vi "SEA_9811_ARINCword2data.vi"(7 "Reverse label bits (F)":bool, 8 "error in (no error)":errorcluster, 10 "timestamp (DBL) in":dbl, 11 "ARINC word in":T2 format="%032b") -> (0 "error out":errorcluster, 3 "ARINC word out":T1 {"ARINC word" format="%032b"})   [LabVIEW 2015]
uses:
  Typdefs/ARINC word.ctl
  Typdefs/ARINC word cluster.ctl
panel:
  out "number":u8 format="%.0o"
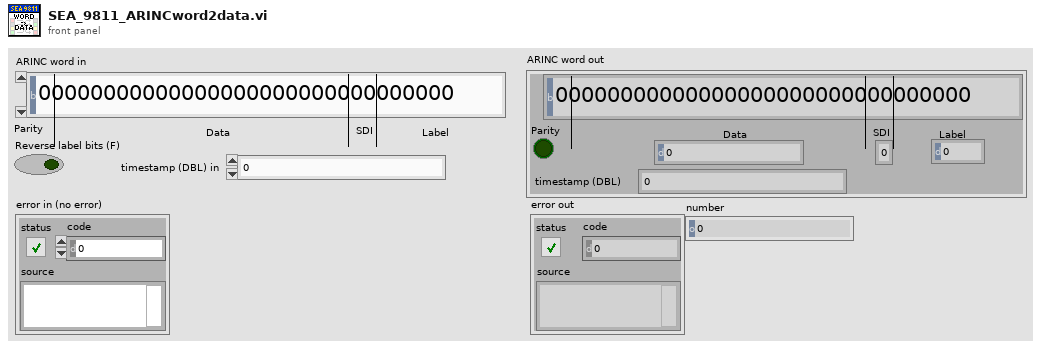
[diagram p1: front panel]
types:
  T1 = typedef "ARINC word cluster.ctl" = cluster{"ARINC word":T2, "Label":u8, "SDI":u8, "Data":u32, "Parity":bool, "timestamp (DBL)":dbl}
  T2 = typedef "ARINC word.ctl" = u32
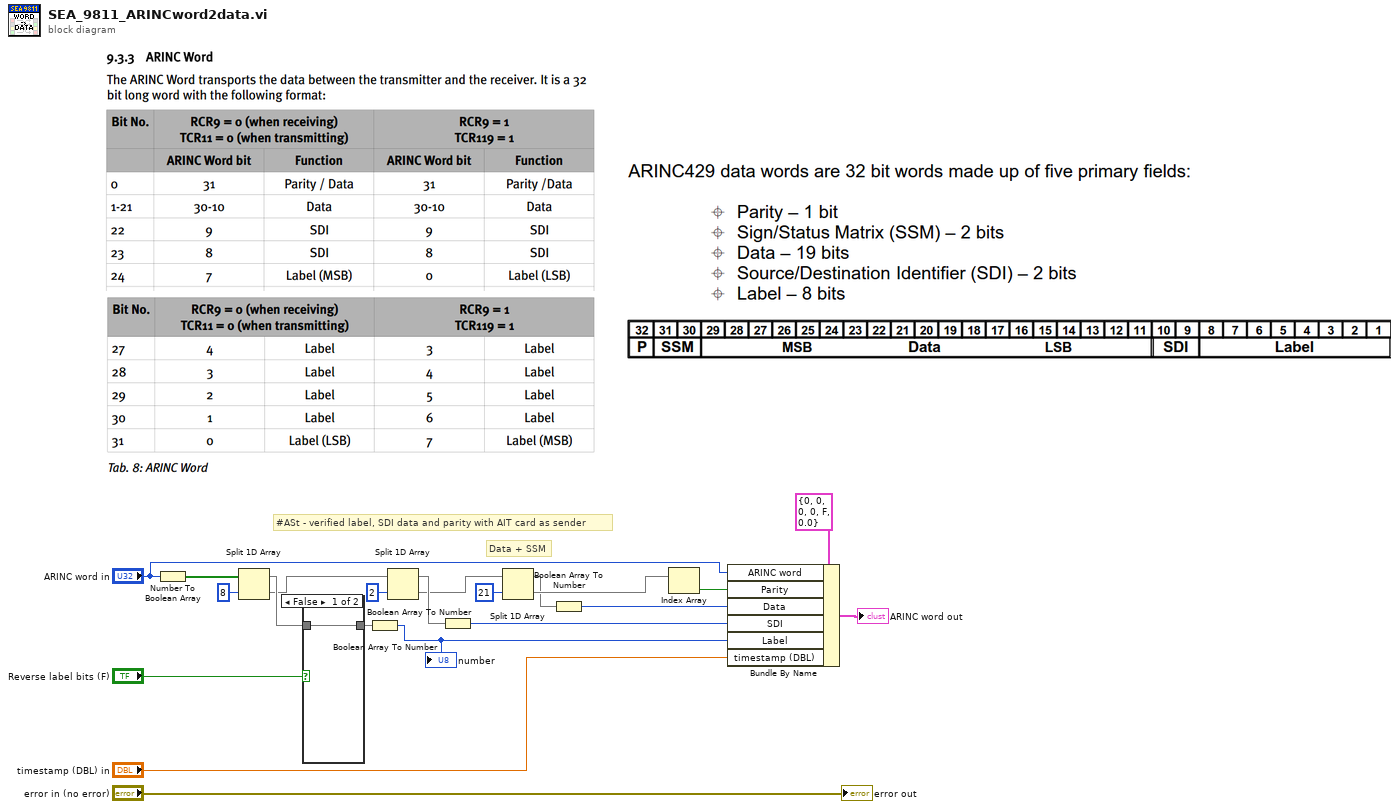
[diagram p0: block diagram]
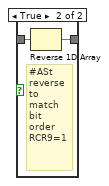
[diagram p2: hidden frame]
diagram:
  # "#ASt - verified label, SDI data and parity with AIT card as sender"
  # "Data + SSM"
  n1 = Number To Boolean Array(number="ARINC word in") -> (Boolean array=w7:bool[])
  n2 = Split 1D Array(array=w7, index=8) -> (first subarray=w6:bool[], second subarray=w5:bool[])
  n3 = case shown="False" "Reverse label bits (F)" {
    tunnel: w6 -> [w22 w24]
    tunnel: [w22 w23] -> w10
    frame False {
    }
    frame True {
      # "#ASt\nreverse\nto \nmatch\nbit\norder\nRCR9=1"
      n4 = Reverse 1D Array(array=w24) -> (reversed array=w23:bool[])
    }
  }
  n5 = Boolean Array To Number(Boolean array=w10) -> (number=w13:u8)
  "number" <- w13
  n6 = Split 1D Array(array=w5, index=2) -> (first subarray=w4:bool[], second subarray=w3:bool[])
  n7 = Boolean Array To Number(Boolean array=w4) -> (number=w14:u8)
  n8 = Split 1D Array(array=w3, index=21) -> (first subarray=w1:bool[], second subarray=w2:bool[])
  n9 = Boolean Array To Number(Boolean array=w1) -> (number=w15:u32)
  n10 = Index Array(array=w2) -> (element=w16:bool)  [unwired: 1 in]
  n11 = Bundle By Name(cluster=T1 {"ARINC word"=0, "Label"=0, "SDI"=0, "Data"=0, "Parity"=FALSE, "timestamp (DBL)"=0.0} ("ARINC word"), "ARINC word"="ARINC word in", "Parity"=w16, "Data"=w15, "SDI"=w14, "Label"=w13, "timestamp (DBL)"="timestamp (DBL) in") -> (→"ARINC word out":T1)
  "error out" <- "error in (no error)"
